vi "Bulk Rename.vi"() -> ()   [LabVIEW 2017]
uses:
  Source/Data Sharing Framework Core/Engine/Transfer Group/Transfer Group.lvclass
panel:
  out "Array 3":string[](array[string])
  out "Array 2":path[](array[path])
  out "Array":path[](array[path])
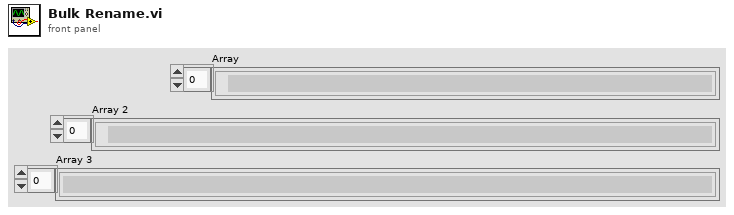
[diagram p1: front panel]
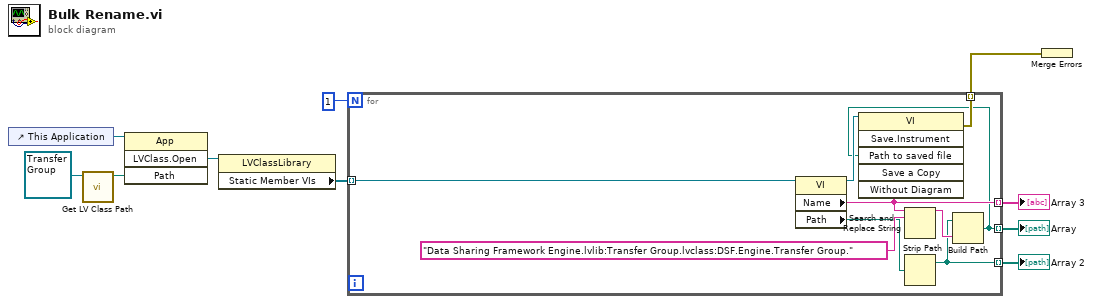
[diagram p0: block diagram]
diagram:
  n1 = control-ref of="This Application"() -> (w10:refnum<vi>)
  n2 = call <vilib>:"Get LV Class Path.vi"("object"=refnum<class "Transfer Group.lvclass"> refnum ("Data Sharing Framework Engine.lvlib:Transfer Group")) -> ("class path"=w9:path)  [unwired: 9 in, 1 out]
  n3 = invoke class="App" method="LVClass.Open"(reference=w10, "Path"=w9) -> ("LVClass.Open"=w7:refnum<vi>)  [unwired: 2 in, 3 out]
  n4 = property class="LVClassLibrary"(reference=w7) -> ("Static Member VIs"=w6:refnum<vi>[])  [unwired: 1 in, 2 out]
  n5 = for {
    N: 1 -> [_]
    tunnel: w6 -> [w19] mode=indexing
    tunnel: [w11] -> w5 mode=indexing
    tunnel: [w15] -> w4 mode=indexing
    tunnel: [w14] -> w3 mode=indexing
    tunnel: [w12] -> w1 mode=indexing
    n6 = property class="VI"(reference=w19) -> (reference out=w13:refnum<vi>, "Name"=w14:string, "Path"=w17:path)  [unwired: 1 in, 1 out]
    n7 = Search and Replace String(input string=w14, search string="Data Sharing Framework Engine.lvlib:Transfer Group.lvclass:DSF.Engine.Transfer Group." ("search string/char (-)")) -> (result string=w16:string)  [unwired: 6 in, 3 out]
    n8 = Strip Path(path=w17) -> (stripped path=w15:path)  [unwired: 1 out]
    n9 = Build Path(base path=w15, name or relative path=w16) -> (appended path=w11:path)
    n10 = invoke class="VI" method="Save.Instrument"(reference=w13, "Path to saved file"=w11) -> (error out=w12:errorcluster)  [unwired: 4 in, 5 out]
  }
  "Array" <- w5
  "Array 2" <- w4
  "Array 3" <- w3
  n11 = Merge Errors(w1) -> ()  [unwired: 1 out]
